vi "DPO.vi"(1 "S":dbl[][](array[numeric]), 2 "x":dbl) -> (0 "y":dbl)   [LabVIEW 2011]
uses:
  <vilib>/imath/engines/lvmath2/RunTimeEngine/ErrorHandling/NIMS_Finalize Error.vi
  <vilib>/imath/engines/lvmath2/RunTimeEngine/BuiltInFunctions/size/NIMS_I32=size(GM,I32).vi
  <instcachedir>/0/NIMS_I32=size(GM,I32)_C888250C35F946008B07D98778967D76.lvgen/NIMS_I32=size(GM,I32)_C888250C35F946008B07D98778967D76_004.vi
  <vilib>/imathl/engines/lvmath/Functions/Error Handling/Create Error.vi
  <vilib>/imath/engines/lvmath2/RunTimeEngine/CommandStatement/NIMS_CommandStatement_MaskErr.vi
  <vilib>/imath/engines/lvmath2/RunTimeEngine/VariableToken/NIMS_VariableToken_CondDefined.vi
  <instcachedir>/0/NIMS_VariableToken_CondDefined_D30D2F4D3CE04567BC79CC35D27951F7.lvgen/NIMS_VariableToken_CondDefined_D30D2F4D3CE04567BC79CC35D27951F7_003.vi
  <vilib>/imath/engines/lvmath/Functions/Error Handling/MergeErrorsWrapper.vi
  <vilib>/imath/engines/lvmath2/RunTimeEngine/NodeEndStatement/NIMS_NodeEndStatement_Output.vi
  <instcachedir>/0/NIMS_NodeEndStatement_Output_53EC0D466D134D7ABD903AC30B43404B.lvgen/NIMS_NodeEndStatement_Output_53EC0D466D134D7ABD903AC30B43404B_001.vi
  <vilib>/imath/engines/lvmath2/RunTimeEngine/CommandStatement/MC_CommandStatement_break.vi
  <vilib>/imath/engines/lvmath2/RunTimeEngine/VariableToken/Read/NIMS_Get Elements - SorM(_,_) - Check - Check(_).vi
  <instcachedir>/0/NIMS_Get Elements - SorM(_,_) - Check - Check(_)_B78B880141DE464ABBC753BC43E627FC.lvgen/NIMS_Get Elements - SorM(_,_) - Check - Check(_)_B78B880141DE464ABBC753BC43E627FC_000.vi
  <vilib>/imath/engines/lvmath2/RunTimeEngine/ErrorHandling/NIMS_Create Error From Enums.vi
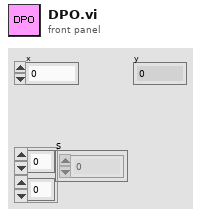
[diagram p1: front panel]
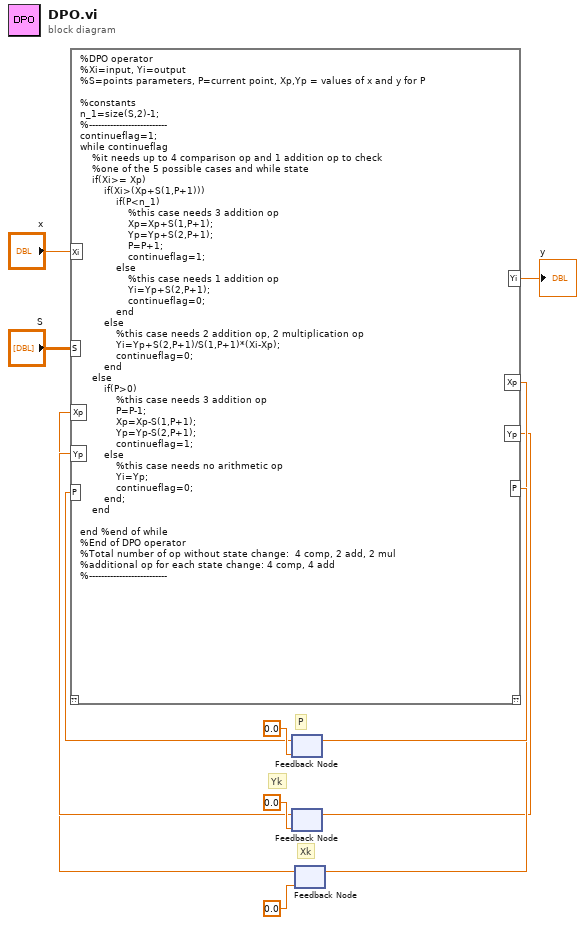
[diagram p0: block diagram]
diagram:
  # "P"
  # "Yk"
  # "Xk"
  n1 = feedback #1(0.0 ("Xk")) -> (w6:dbl)
  n2 = feedback #2(0.0 ("Xk")) -> (w10:dbl)
  n3 = feedback #3(0.0 ("Xk")) -> (w3:dbl)
  n4 = mathscript code="%DPO operator\n%Xi=input, Yi=output\n%S=points parameters, P=current point, Xp,Yp = values of x and y for P\n\n%constants\nn_1=size(S,2)-1;\n%--------------------------\ncontinueflag=1;\nwhile continueflag\n    %it needs up to 4 comparison op and 1 addition op to check\n    %one of the 5 possible cases and while state\n    if(Xi>= Xp)   \n        if(Xi>(Xp+S(1,P+1)))                                               \n            if(P<n_1)\n                %this case needs 3 addition op\n                Xp=Xp+S(1,P+1);\n                Yp=Yp+S(2,P+1);\n                P=P+1;  \n                continueflag=1;\n            else\n                %this case needs 1 addition op\n                Yi=Yp+S(2,P+1);\n                continueflag=0;\n            end             \n        else\n            %this case needs 2 addition op, 2 multiplication op\n            Yi=Yp+S(2,P+1)/S(1,P+1)*(Xi-Xp);\n            continueflag=0;\n        end\n    else\n        if(P>0)\n            %this case needs 3 addition op\n            P=P-1;                    \n            Xp=Xp-S(1,P+1);\n            Yp=Yp-S(2,P+1);\n            continueflag=1;\n        else\n            %this case needs no arithmetic op\n            Yi=Yp;\n            continueflag=0;\n        end;\n    end\n\nend %end of while\n%End of DPO operator\n%Total number of op without state change:  4 comp, 2 add, 2 mul\n%additional op for each state change: 4 comp, 4 add\n%--------------------------"("Xi"="x", "Yp"=w10, "P"=w6, "S"="S", "Xp"=w3) -> ("P"=w8:dbl, "Yi"=→"y":dbl, "Xp"=w4:dbl, "Yp"=w2:dbl)  [unwired: 1 in, 1 out]
  n5 = feedback-in #1(w8) -> ()
  n6 = feedback-in #2(w2) -> ()
  n7 = feedback-in #3(w4) -> ()
